vi "YTicks0006.vi"   [LabVIEW 2013]
uses:
  ModeType.ctl
  <vilib>/Heliosphere Research LLC/Advanced Plotting Toolkit/api_core/NewPlotScales.ctl
  ErrorCodes.ctl
  <vilib>/Heliosphere Research LLC/Advanced Plotting Toolkit/Advanced Plotting Toolkit.lvlib
types:
  T1 = typedef "ErrorCodes.ctl" = u32
  T2 = typedef "Advanced Plotting Toolkit.lvlib/NewPlotScales.ctl" = enum16{"Default", "Linear", "Log", "Symlog"}
  T3 = typedef "ModeType.ctl" = enum16{"Normal", "Expected Failure", "Skipped", "Broken"}
  T4 = typedef "Advanced Plotting Toolkit.lvlib/PlotID.ctl" = i32
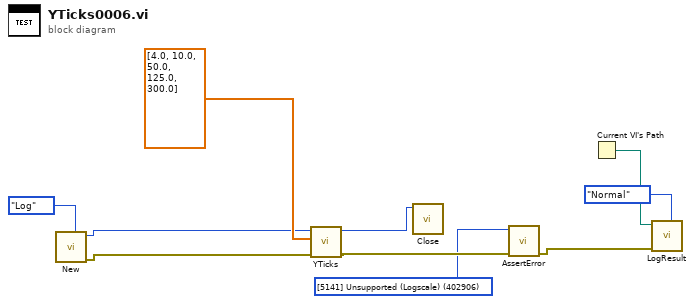
[diagram p0: block diagram]
diagram:
  w1 = T1 402906 items=["[5120] Invalid ID"=402902, "[5110] Failed to Init"=402900, "[5111] Unknown Error"=402901, "[5130] Save - Bad File Extension"=402403, "[5131] Save - General Error"=402904, "[5140] Unsupported (Polar)"=402905, "[5141] Unsupported (Logscale)"=402906, "[5142] Coordinates Not Regular"=402907] ("Expected Error")
  n1 = call <vilib>:"New.vi"("Y Axis Scale"=NewPlotScales."Log") -> ("error out"=w5:errorcluster, "Plot ID"=w6:T4)  [unwired: 9 in]
  n2 = call <vilib>:"YTicks.vi"("error in (no error)"=w5, "Tick Locations"=dbl[] [4.0, 10.0, 50.0, 125.0, 300.0], "Plot ID"=w6) -> ("error out"=w4:errorcluster, "Plot ID Out"=w3:T4)  [unwired: 7 in]
  n3 = call <vilib>:"Close.vi"("Plot ID"=w3) -> ()  [unwired: 10 in, 1 out]
  n4 = call "AssertError.vi"("error in (no error)"=w4, "Expected Error"=w1) -> ("error out"=w2:errorcluster)  [unwired: 9 in]
  n5 = Current VI's Path() -> (path=w10:path)
  n6 = call "LogResult.vi"("Mode"=ModeType."Normal", "Test Result"=w2, "VI Path"=w10) -> ()  [unwired: 9 in]
